vi "Children Content.vi"(7 "Context":refnum<class "Context.lvclass">, 8 "Error In":errorcluster, 11 "Section In":refnum<class "Section.lvclass">) -> (0 "Error Out":errorcluster, 2 "Content":string, 3 "Section Out":refnum<class "Section.lvclass">)   [LabVIEW 2018, in "Toolkit.lvlib" / "Nodes.lvlib" / "Section.lvclass"]
uses:
  Section.lvclass
  Data/Context/Context.lvclass
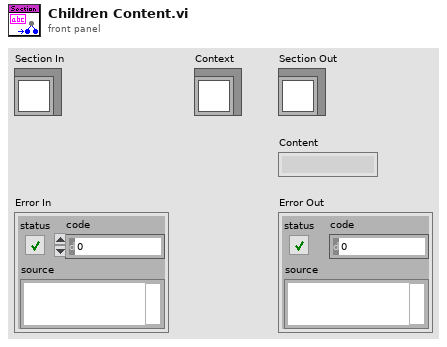
[diagram p1: front panel]
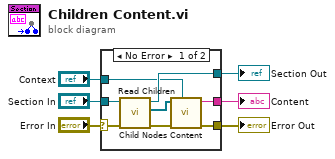
[diagram p0: block diagram]
diagram:
  n1 = case shown="No Error" "Error In" {
    selector: "Error In" -> [w9 w15]
    tunnel: [w14 _] -> w6
    tunnel: [w13 w15] -> w5
    tunnel: "Context" -> [w7 _]
    tunnel: [w11 w16] -> w3
    tunnel: "Section In" -> [w10 w16]
    frame No Error {
      n2 = call-dynamic "Read Children.vi"("Error In"=w9, "NonTerminal In"=w10) -> ("Error Out"=w12:errorcluster, "Children"=w8:refnum<class "Abstract.lvclass">[], "NonTerminal Out"=w11:refnum<class "Section.lvclass">)  [unwired: 7 in]
      n3 = call "Child Nodes Content.vi"("Context"=w7, "Error In"=w12, "Children"=w8) -> ("Error Out"=w13:errorcluster, "Content"=w14:string)  [unwired: 7 in]
    }
    frame Error {
    }
  }
  "Content" <- w6
  "Error Out" <- w5
  "Section Out" <- w3
